vi "AnemoToString.vi"(11 "Normal,Crossflow":dbl[](array[numeric])) -> (1 "Theta":string, 2 "Vmag":string, 3 "Normal,Crossflow":string[](array[string]))   [LabVIEW 2016]
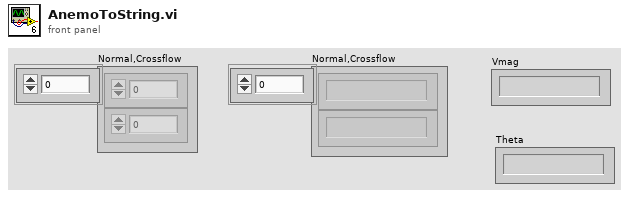
[diagram p1: front panel]
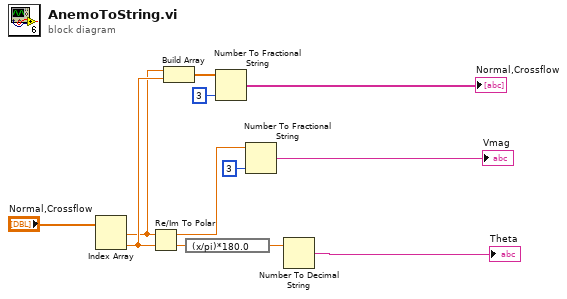
[diagram p0: block diagram]
diagram:
  n1 = Index Array(array="Normal,Crossflow") -> (element #1=w2:dbl, element #2=w3:dbl)  [unwired: 2 in]
  n2 = Re/Im To Polar(2:w3, 3:w2) -> (0:w4:dbl, 1:w8:dbl)
  n3 = Build Array(w2, w3) -> (w6:dbl[])
  n4 = expression code="(x/pi)*180.0" ("radians to degrees")(w4) -> (w9:dbl)
  n5 = Number To Fractional String(number=w6, precision (6)=i16 3) -> (F-format string=→"Normal,Crossflow":string[])  [unwired: 2 in]
  n6 = Number To Fractional String(number=w8, precision (6)=i16 3) -> (F-format string=→"Vmag":string)  [unwired: 2 in]
  n7 = Number To Decimal String(number=w9) -> (decimal integer string=→"Theta":string)  [unwired: 1 in]
